vi "write primary network adapter.vi"(8 "error in":errorcluster, 10 "network adapter settings":T1={"IP address"="", "MAC address"="", "IP address request mode"=1, "subnet mask"="", "gateway"="", "DNS server"="", "adapter mode"=1, "adapter type"=1} {"IP address request mode" items=["Static"=1, "DHCP/Link Local"=2, "Link-Local Only"=4, "DHCP Only"=8]; "adapter type" items=["Ethernet"=1, "WLAN"=2]; "adapter mode" items=["Disabled"=1, "TCP/IP Ethernet"=2, "Deterministic"=4, "EtherCAT"=8, "TCP/IP WLAN Connect"=32, "TCP/IP WLAN Create"=64]}, 11 "controller in":refnum<class "Controller.lvclass">) -> (0 "error out":errorcluster, 3 "controller out":refnum<class "Controller.lvclass">)   [LabVIEW 2014, in "SMI.lvlib" / "Controller.lvclass"]
uses:
  Controller.lvclass
  network adapter settings.ctl
  Controller.lvclass/Controller.ctl
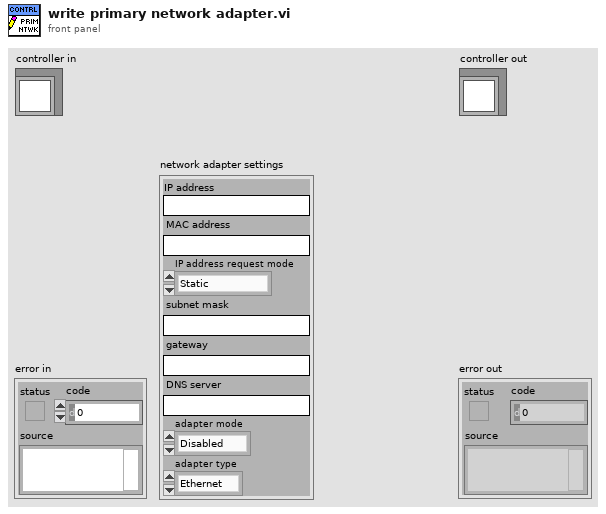
[diagram p1: front panel]
types:
  T1 = typedef "SMI.lvlib/Controller.lvclass/network adapter settings.ctl" = cluster{"IP address":string, "MAC address":string, "IP address request mode":u32, "subnet mask":string, "gateway":string, "DNS server":string, "adapter mode":u32, "adapter type":u32}
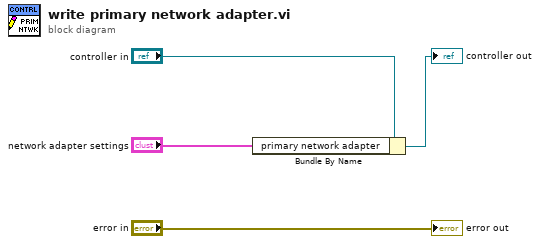
[diagram p0: block diagram]
diagram:
  n1 = Bundle By Name(cluster="controller in", "primary network adapter"="network adapter settings") -> (→"controller out":refnum<class "Controller.lvclass">)
  "error out" <- "error in"
